vi "Configure Measurement.vi"(6 "Manual Resolution (10 PLC)":u16(ring)=9 items=["0.001 PLC", "0.006 PLC", "0.02 PLC", "0.06 PLC", "0.2 PLC", "0.6 PLC", "1 PLC", "2 PLC", "3 HZ", "10 PLC", "20 HZ", "100 PLC", "200 HZ"], 7 "Manual Range ( 1.0)":dbl=1.0, 8 "error in (no error)":errorcluster, 9 "Enable Auto Range ( T:Enable)":bool=TRUE, 10 "Function ( 0:DC Voltage)":u16(ring) items=["DC Voltage", "AC Voltage", "DC Current", "AC Current", "2W Resistance", "4W Resistance", "Frequency", "Period", "Continuity", "Diode", "VDC Ratio", "Temperature", "TCouple", "Capacitance"], 11 "VISA Resource Name":refnum<visa-resource-name>) -> (0 "error out":errorcluster, 3 "VISA resource name out":refnum<visa-resource-name>)   [LabVIEW 2020, in "PICOTEST M351XA Series.lvlib"]
doc: "Configures the measurement type, resolution, and range on the instrument.\n\n<B>Note:</B>\n\nThis VI must be called before other configuration VIs."
uses:
  PICOTEST M351XA Series.lvlib
panel:
  # "To avoid the value of Range and Resolution\nout of range,please see the \"Description and\nTip\" first before you input it.The Picotest\nM3511A does not support TCouple Function."
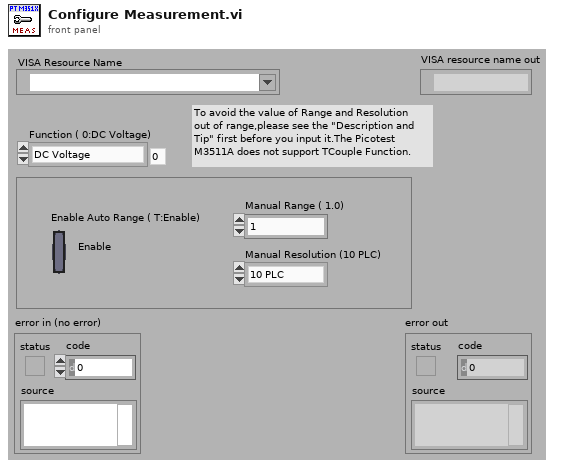
[diagram p1: front panel]
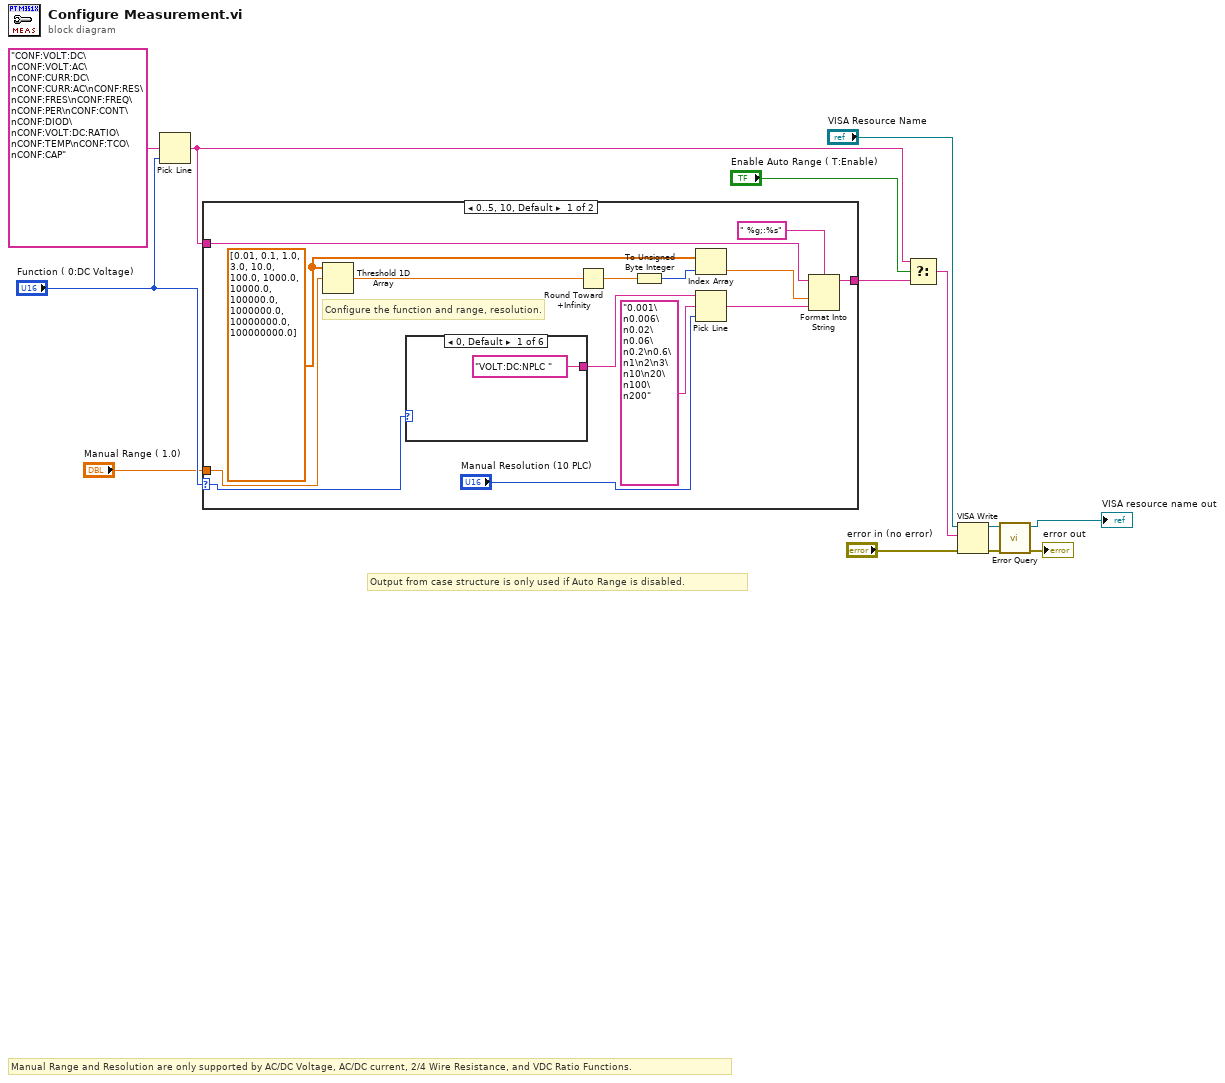
[diagram p0: block diagram]
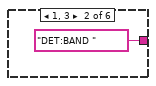
[diagram p2: hidden frame]
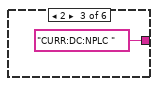
[diagram p3: hidden frame]
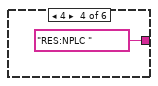
[diagram p4: hidden frame]
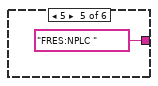
[diagram p5: hidden frame]
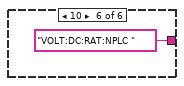
[diagram p6: hidden frame]
diagram:
  # "Output from case structure is only used if Auto Range is disabled."
  # "Manual Range and Resolution are only supported by AC/DC Voltage, AC/DC current, 2/4 Wire Resistance, and VDC Ratio Functions."
  n1 = Pick Line(multi-line string="CONF:VOLT:DC\nCONF:VOLT:AC\nCONF:CURR:DC\nCONF:CURR:AC\nCONF:RES\nCONF:FRES\nCONF:FREQ\nCONF:PER\nCONF:CONT\nCONF:DIOD\nCONF:VOLT:DC:RATIO\nCONF:TEMP\nCONF:TCO\nCONF:CAP", line index="Function ( 0:DC Voltage)") -> (output string=w5:string)  [unwired: 1 in]
  n2 = case shown="0..5, 10, Default" "Function ( 0:DC Voltage)" {
    selector: "Function ( 0:DC Voltage)" -> [w14 _]
    tunnel: w5 -> [w27 w34]
    tunnel: [w26 w34] -> w12
    tunnel: "Manual Range ( 1.0)" -> [w25 _]
    frame 0..5, 10, Default {
      w23 = dbl[] [0.01, 0.1, 1.0, 3.0, 10.0, 100.0, 1000.0, 10000.0, 100000.0, 1000000.0, 10000000.0, 100000000.0]
      # "Configure the function and range, resolution."
      n3 = Threshold 1D Array(2:w25, 3:w23) -> (0:w24:dbl)  [unwired: 1 in]
      n4 = case shown="0, Default" w14 {
        tunnel: ["VOLT:DC:NPLC " "DET:BAND " "CURR:DC:NPLC " "RES:NPLC " "FRES:NPLC " "VOLT:DC:RAT:NPLC "] -> w16
        frame 0, Default {
        }
        frame 1, 3 {
        }
        frame 2 {
        }
        frame 4 {
        }
        frame 5 {
        }
        frame 10 {
        }
      }
      n5 = Round Toward +Infinity(x=w24) -> (ceil(x): smallest int >= x=w22:dbl)
      n6 = To Unsigned Byte Integer(number=w22) -> (unsigned 8bit integer=w21:u8)
      n7 = Index Array(array=w23, index=w21) -> (element=w20:dbl)
      n8 = Pick Line(string ("")=w16, multi-line string="0.001\n0.006\n0.02\n0.06\n0.2\n0.6\n1\n2\n3\n10\n20\n100\n200", line index="Manual Resolution (10 PLC)") -> (output string=w18:string)
      n9 = Format Into String(format string=" %g;:%s", initial string=w27, w20, w18) -> (resulting string=w26:string)  [unwired: 1 in, 1 out]
    }
    frame 6..9, 11..13 {
      # "Manual range & resolution are not supported by these functions:\n6: Frequency\n7: Period\n8: Continuity\n9: Diode\n11: Temperature\n12: TCouple \n13: Capacitance"
    }
  }
  n10 = Select(t=w5, s="Enable Auto Range ( T:Enable)", f=w12) -> (s? t:f=w8:string)
  n11 = VISA Write(VISA resource name="VISA Resource Name", write buffer=w8, error in (no error)="error in (no error)") -> (VISA resource name out=w4:refnum<visa-resource-name>, error out=w3:errorcluster)  [unwired: 1 out]
  n12 = call "Error Query.vi"("error in (no error)"=w3, "VISA resource name"=w4) -> ("error out"=→"error out":errorcluster, "VISA resource name out"=→"VISA resource name out":refnum<visa-resource-name>)  [unwired: 6 in, 2 out]
